vi "Get CLAP Data.vi"(11 "CLAP in":refnum<class "CLAP.lvclass">) -> (0 "error out":errorcluster, 3 "CLAP out":refnum<class "CLAP.lvclass">)   [LabVIEW 2012]
uses:
  Devices/CLAP/CLAP.lvclass
  Reusable/Serial IO/Read - Asynchronous.vi
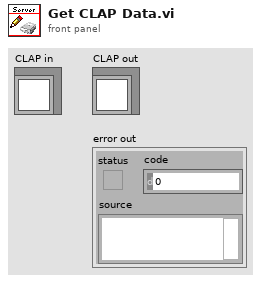
[diagram p1: front panel]
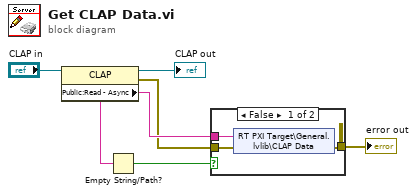
[diagram p0: block diagram]
diagram:
  n1 = property class="CLAP"(reference="CLAP in") -> (reference out=→"CLAP out":refnum<class "CLAP.lvclass">, error out=w1:errorcluster, "Public:Read - Async"=w5:string)  [unwired: 1 in]
  n2 = Empty String/Path?(string/path=w5) -> (empty?=w4:bool)
  n3 = case shown="False" w4 {
    tunnel: w1 -> [w9 w10]
    tunnel: w5 -> [w8 _]
    tunnel: [w7 w10] -> w6
    frame False {
      n4 = shared-variable "RT PXI Target\\General.lvlib\\CLAP Data"(w8, error in=w9) -> (error out=w7:errorcluster)
    }
    frame True {
    }
  }
  "error out" <- w6
